vi "Handle Command.vi"(8 "error in (no error)":errorcluster, 9 "Value":bool, 11 "Valve in":refnum<class "HitAndHoldControl.lvclass">) -> (0 "error out":errorcluster, 3 "Valve out":refnum<class "HitAndHoldControl.lvclass">)   [LabVIEW 2020, in "VolatusControl.lvlib" / "HitAndHoldControl.lvclass"]
uses:
  HitAndHoldControl.lvclass
  HitAndHoldControl.lvclass/HitAndHoldControl.ctl
  HitAndHold State.ctl
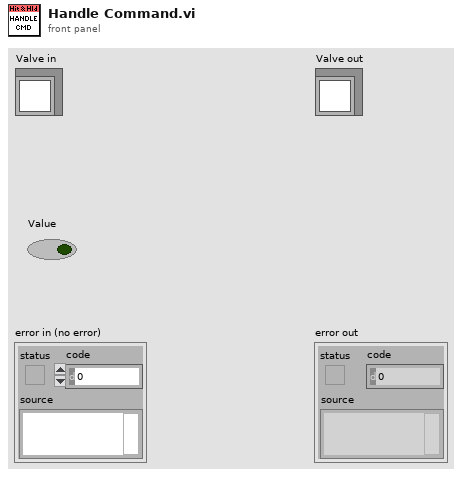
[diagram p1: front panel]
types:
  T1 = typedef "VolatusControl.lvlib/HitAndHoldControl.lvclass/HitAndHold State.ctl" = enum16{"Idle", "Hit", "Dwell", "Hold", "Off"}
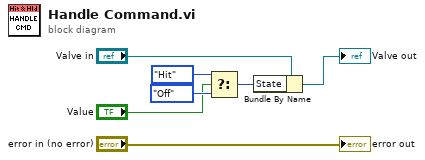
[diagram p0: block diagram]
diagram:
  n1 = Select(t=HitAndHold_State."Hit" ("State"), s="Value", f=HitAndHold_State."Off" ("State")) -> (s? t:f=w1:T1)
  n2 = Bundle By Name(cluster="Valve in", "State"=w1) -> (→"Valve out":refnum<class "HitAndHoldControl.lvclass">)
  "error out" <- "error in (no error)"
